vi "Search DQMH Module name from selection.vi"(11 "Search Module Name":string="\\Panther Dashboard for DQMH.lvproj\\Coins.lvlib\\Broadcast\\Error Reported") -> (3 "Module Name":string)   [LabVIEW 2020, in "Panther Dashboard.lvlib"]
uses:
  Panther Dashboard.lvlib
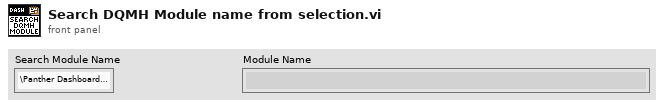
[diagram p1: front panel]
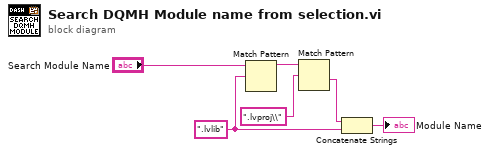
[diagram p0: block diagram]
diagram:
  w3 = ".lvlib" ("regular expression")
  n1 = Match Pattern(string="Search Module Name", regular expression=w3) -> (before substring=w5:string)  [unwired: 1 in, 3 out]
  n2 = Match Pattern(string=w5, regular expression=".lvproj\\") -> (after substring=w2:string)  [unwired: 1 in, 3 out]
  n3 = Concatenate Strings(w2, w3) -> (→"Module Name":string)
